vi "sv_Refresh for Octave.vi"(4 "axes IN":T1 {"y axis maximum" format="%.2f"; "y axis minimum" format="%.2f"; "z axis maximum" format="%.2f"; "z axis minimum" format="%.2f"; "x axis maximum" format="%.2f"; "x axis minimum" format="%.2f"; "z axis height [%]" format="%.2f"; "x axis width [%]" format="%.2f"}, 5 "event queue IN":string[](array[string])) -> (0 "clear graph?":bool, 1 "axes OUT":T1 {"y axis maximum" format="%.2f"; "y axis minimum" format="%.2f"; "z axis maximum" format="%.2f"; "z axis minimum" format="%.2f"; "x axis maximum" format="%.2f"; "x axis minimum" format="%.2f"; "z axis height [%]" format="%.2f"; "x axis width [%]" format="%.2f"}, 2 "event queue OUT":string[](array[string]))   [LabVIEW 2017]
uses:
  <vilib>/addons/Sound and Vibration/compatibility/Waterfall/subVIs/sv_Waterfall for Octave Global.vi
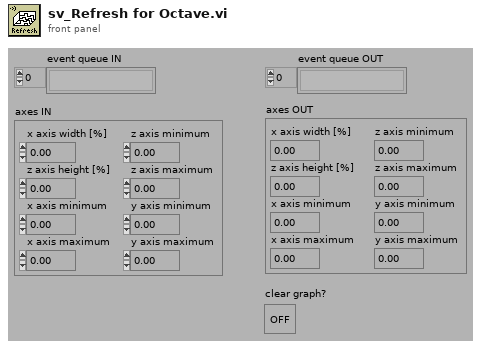
[diagram p1: front panel]
types:
  T1 = cluster{"x axis width [%]":dbl, "z axis height [%]":dbl, "x axis minimum":dbl, "x axis maximum":dbl, "z axis minimum":dbl, "z axis maximum":dbl, "y axis minimum":dbl, "y axis maximum":dbl}
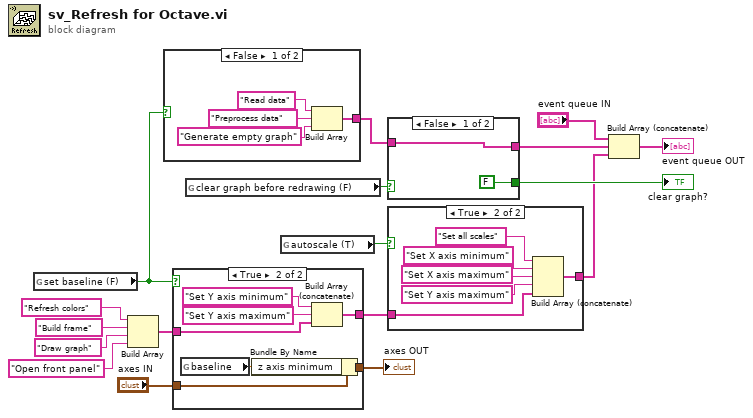
[diagram p0: block diagram]
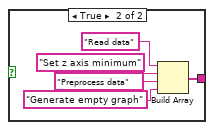
[diagram p3: hidden frame]
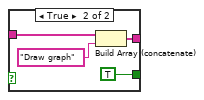
[diagram p5: hidden frame]
diagram:
  n1 = global read "sv_Waterfall for Octave Global.vi" "set baseline (F)"() -> (w7:bool)
  n2 = Build Array("Refresh colors", "Build frame", "Draw graph", "Open front panel") -> (w11:string[])
  n3 = case shown="False" w7 {
    tunnel: [w18 w22] -> w12
    frame False {
      n4 = Build Array("Read data", "Preprocess data", "Generate empty graph") -> (w18:string[])
    }
    frame True {
      n5 = Build Array("Read data", "Set z axis minimum", "Preprocess data", "Generate empty graph") -> (w22:string[])
    }
  }
  n6 = case shown="True" w7 {
    tunnel: w11 -> [w28 w32]
    tunnel: [w28 w33] -> w10
    tunnel: "axes IN" -> [w27 w31]
    tunnel: [w27 w30] -> w8
    frame False {
    }
    frame True {
      n7 = global read "sv_Waterfall for Octave Global.vi" "baseline"() -> (w29:dbl)
      n8 = Bundle By Name(cluster=w31, "z axis minimum"=w29) -> (w30:T1)
      n9 = Build Array (concatenate)("Set Y axis minimum", "Set Y axis maximum", w32) -> (w33:string[])
    }
  }
  "axes OUT" <- w8
  n10 = global read "sv_Waterfall for Octave Global.vi" "clear graph before redrawing (F)"() -> (w5:bool)
  n11 = global read "sv_Waterfall for Octave Global.vi" "autoscale (T)"() -> (w6:bool)
  n12 = case shown="False" w5 {
    tunnel: [FALSE TRUE] -> w17
    tunnel: w12 -> [w37 w40]
    tunnel: [w37 w38] -> w14
    frame False {
    }
    frame True {
      n13 = Build Array (concatenate)(w40, "Draw graph") -> (w38:string[])
    }
  }
  "clear graph?" <- w17
  n14 = case shown="True" w6 {
    tunnel: [w42 w43] -> w9
    tunnel: w10 -> [w42 w44]
    frame False {
    }
    frame True {
      n15 = Build Array (concatenate)("Set all scales", "Set X axis minimum", "Set X axis maximum", "Set Y axis maximum", w44) -> (w43:string[])
    }
  }
  n16 = Build Array (concatenate)("event queue IN", w14, w9) -> (→"event queue OUT":string[])
